vi "SETI_Host_Interface.vi"() -> ()   [LabVIEW 2015]
uses:
  SETI FPGA States.ctl
  <vilib>/rvi/Emulation/niFpgaGetClockAttributes.vi
  <vilib>/rvi/Emulation/niFpgaSctlEmulationGetInTimedLoop.vi
  <vilib>/rvi/Emulation/niFpgaEmulationReportErrorSimple.vi
  <vilib>/rvi/Emulation/niFpgaProcessEmulError.vi
  <vilib>/rvi/interface/RandomDataEmulation/niFpgaRandomDataHandleErrors.vi
  <vilib>/rvi/Emulation/niFpgaCriticalErrorInLSC.vi
  <vilib>/rvi/DataTransferAndStorage/Container/XNode/niFpgaContainer.xnode
  <vilib>/rvi/interface/RandomDataEmulation/nirviRandomDataFpgaReadWriteTemplate.vi
panel:
  out "FPGA Loop Count":i32
  out "State":T1
  out "Total":u64
  out "Count":i32
  in  "Number of Data Points":i16
  in  "Start":bool
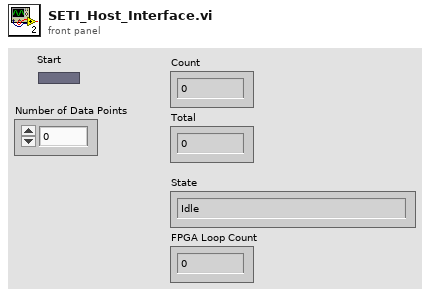
[diagram p1: front panel]
types:
  T1 = typedef "SETI FPGA States.ctl" = enum16{"Idle", "GetNumPoints", "GetChirpRate", "Process", "Stop"}
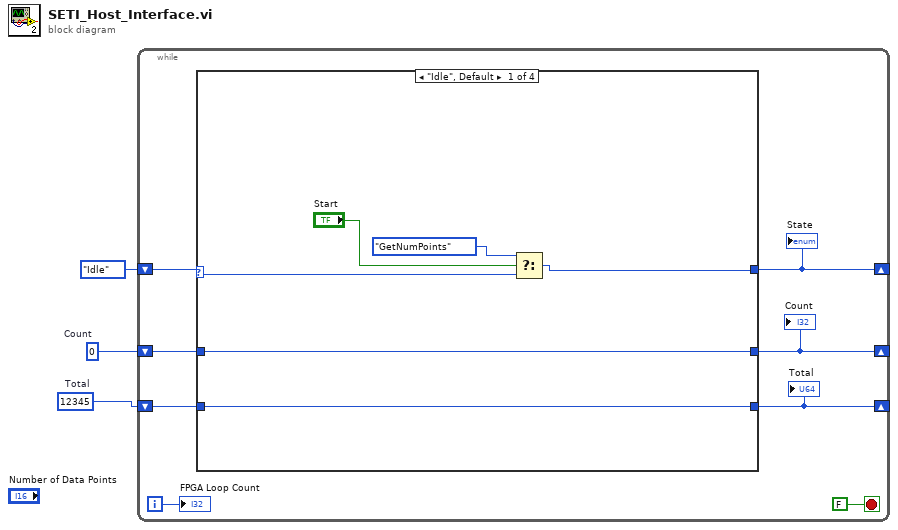
[diagram p0: block diagram]
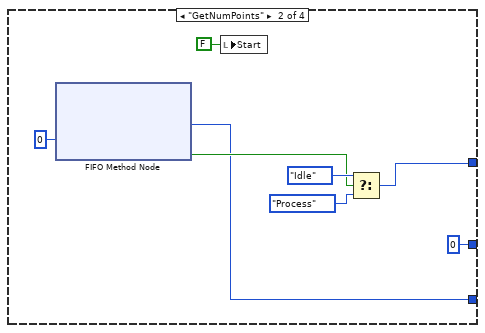
[diagram p2: hidden frame]
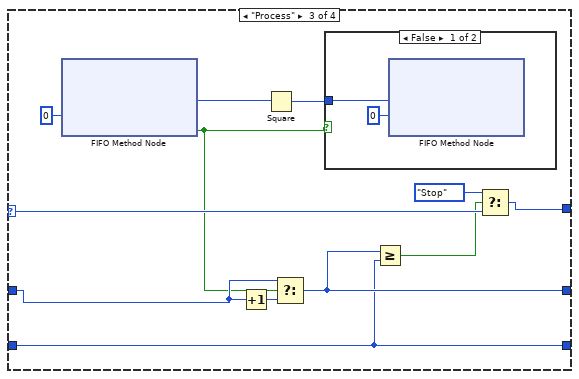
[diagram p3: hidden frame]
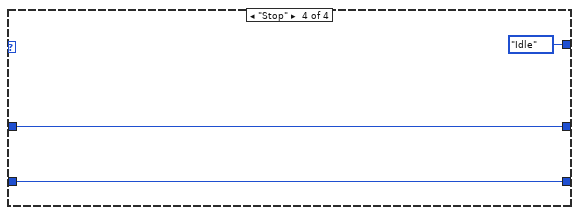
[diagram p5: hidden frame]
diagram:
  w1 = u64 12345  # Total
  w2 = 0  # Count
  n1 = while {
    shift-right: [w10] -> _
    shift-left: SETI_FPGA_States."Idle" -> [w11]
    shift-right: [w7] -> _
    shift-left: w2 -> [w8]
    shift-right: [w5] -> _
    shift-left: w1 -> [w6]
    i -> [w4]
    stop <- FALSE stop-if-true
    n2 = case shown="\"Idle\", Default" w11 {
      selector: w11 -> [w16 _ w33 _]
      tunnel: [w15 w19 w32 SETI_FPGA_States."Idle"] -> w10
      tunnel: w8 -> [w13 _ w34 w41]
      tunnel: [w13 0 ("Timeout") w28 w41] -> w7
      tunnel: w6 -> [w12 _ w27 w40]
      tunnel: [w12 w18 w27 w40] -> w5
      frame "Idle", Default {
        n3 = Select(t=SETI_FPGA_States."GetNumPoints", s="Start", f=w16) -> (s? t:f=w15:T1)
      }
      frame "GetNumPoints" {
        n4 = xnode ("FIFO Method Node")("Timeout"=0) -> ("Element"=w18:u64, "Timed Out?"=w21:bool)  [unwired: 1 in, 1 out]
        n5 = local write "Start"(FALSE ("Start")) -> ()
        n6 = Select(t=SETI_FPGA_States."Idle", s=w21, f=SETI_FPGA_States."Process") -> (s? t:f=w19:T1)
      }
      frame "Process" {
        n7 = xnode ("FIFO Method Node")("Timeout"=0) -> ("Element"=w37:u64, "Timed Out?"=w26:bool)  [unwired: 1 in, 1 out]
        n8 = Increment(x=w34) -> (x+1=w29:i32)
        n9 = Square(x=w37) -> (x^2=w36:u64)
        n10 = Select(t=w34, s=w26, f=w29) -> (s? t:f=w28:i32)
        n11 = case shown="False" w26 {
          tunnel: w36 -> [w39 _]
          frame False {
            n12 = xnode ("FIFO Method Node")("Element"=w39, "Timeout"=0) -> ()  [unwired: 1 in, 2 out]
          }
          frame True {
          }
        }
        n13 = Greater Or Equal?(x=w28, y=w27) -> (x >= y?=w31:bool)
        n14 = Select(t=SETI_FPGA_States."Stop", s=w31, f=w33) -> (s? t:f=w32:T1)
      }
      frame "Stop" {
      }
    }
    "Count" <- w7
    "Total" <- w5
    "State" <- w10
    "FPGA Loop Count" <- w4
  }
